vi "pass new incidents onto the network stream.vi"(7 "RT Queues":T1, 8 "Comms data":T2={"Parameters"={"error writer name"="error writer", "command reader name"="command reader", "error buffer size"=16, "command buffer size"=16, "scanivalveIP"="", "scanivalvePeriod"=16}, "Variables"={"listen schedule"=0, "incident buffer"=[], "command stream"="", "error stream"="", "waiting for command stream connect"=FALSE, "waiting for error stream connect"=FALSE, "scanivalve connection"=refnum, "scanivalveScheduleID"=16}}, 10 "incident":variant) -> (0 "Comms data out":T2={"Parameters"={"error writer name"="error writer", "command reader name"="command reader", "error buffer size"=16, "command buffer size"=16, "scanivalveIP"="", "scanivalvePeriod"=16}, "Variables"={"listen schedule"=0, "incident buffer"=[], "command stream"="", "error stream"="", "waiting for command stream connect"=FALSE, "waiting for error stream connect"=FALSE, "scanivalve connection"=refnum, "scanivalveScheduleID"=16}}, 2 "buffered messages":i32)   [LabVIEW 2018]
uses:
  comms data.ctl
  Type Defs/generic incident.ctl
  Type Defs/Queues cluster.ctl
  Chris VIs/Message Scheduler/message scheduler.lvclass
  Queue VIs/En-queue RT comms element.vi
  <resource>/objmgr/ni.dex.rc
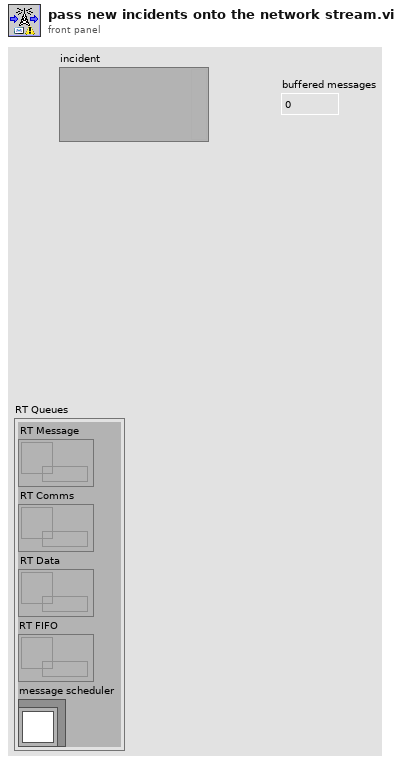
[diagram p1: front panel]
types:
  T1 = typedef "Queues cluster.ctl" = cluster{"RT Message":refnum<queue>, "RT Comms":refnum<queue>, "RT Data":refnum<queue>, "RT FIFO":refnum<queue>, "message scheduler":refnum<class "message scheduler.lvclass">}
  T2 = typedef "comms data.ctl" = cluster{"Parameters":cluster{"error writer name":string, "command reader name":string, "error buffer size":i32, "command buffer size":i32, "scanivalveIP":string, "scanivalvePeriod":u16}, "Variables":cluster{"listen schedule":u32, "incident buffer":T3[], "command stream":refnum<k21>, "error stream":refnum<k21>, "waiting for command stream connect":bool, "waiting for error stream connect":bool, "scanivalve connection":refnum<k5>, "scanivalveScheduleID":u32}}
  T3 = typedef "generic incident.ctl" = cluster{"timestamp":timestamp, "type":string, "Variant":variant}
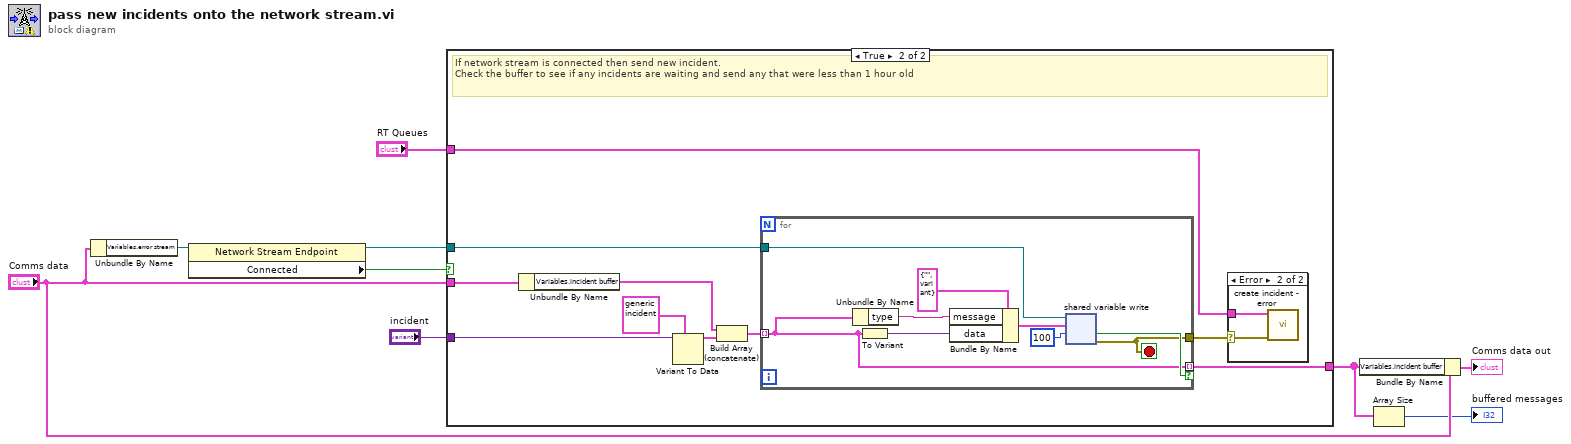
[diagram p0: block diagram]
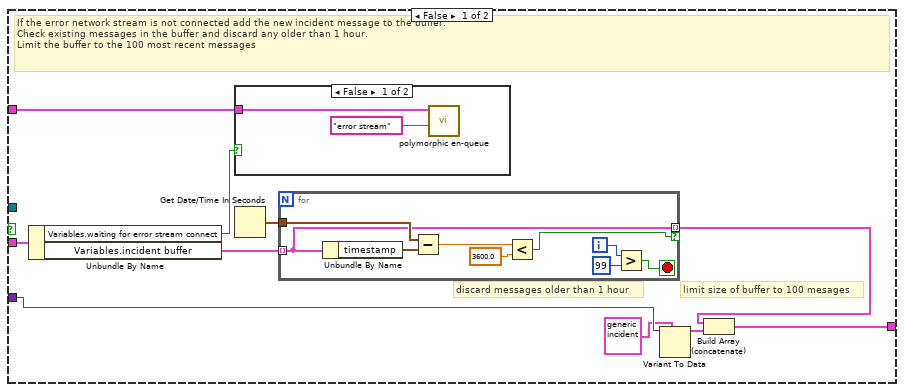
[diagram p2: hidden frame]
diagram:
  n1 = Unbundle By Name("Comms data") -> ("Variables.error stream"=w9:refnum<k21>)
  n2 = property class="Network Stream Endpoint"(reference=w9) -> (reference out=w8:refnum<k21>, "Connected"=w7:bool)  [unwired: 1 in, 1 out]
  n3 = case shown="True" w7 {
    tunnel: w8 -> [_ w34]
    tunnel: "incident" -> [w16 w39]
    tunnel: "Comms data" -> [w18 w40]
    tunnel: [w12 w33] -> w2
    tunnel: "RT Queues" -> [w11 w31]
    frame False {
      # "discard messages older than 1 hour"
      # "limit size of buffer to 100 mesages"
      # "If the error network stream is not connected add the new incident message to the buffer.\nCheck existing messages in the buffer and discard any older than 1 hour.\nLimit the buffer to the 100 most recent messages"
      n4 = Unbundle By Name(w18) -> ("Variables.waiting for error stream connect"=w10:bool, "Variables.incident buffer"=w17:T3[])
      n5 = case shown="False" w10 {
        tunnel: w11 -> [w21 _]
        frame False {
          n6 = call-poly "polymorphic en-queue.vi"("Message"="error stream", "RT Queues"=w21) -> ()  [unwired: 9 in, 1 out]
        }
        frame True {
        }
      }
      n7 = Get Date/Time In Seconds() -> (seconds since 1Jan1904=w19:timestamp)
      n8 = for {
        tunnel: w19 -> [w28]
        tunnel: w17 -> [w23] mode=indexing
        tunnel: [w23] -> w13 mode=indexing if=w22
        i -> [w27]
        stop <- w25 stop-if-true
        n9 = Unbundle By Name(w23) -> ("timestamp"=w24:timestamp)
        n10 = Subtract(x=w28, y=w24) -> (x-y=w30:dbl)
        n11 = Less?(x=w30, y=3600.0) -> (x < y?=w22:bool)
        n12 = Greater?(x=w27, y=99) -> (0:w25:bool)
      }
      n13 = Variant To Data(type=T3 {"timestamp"=timestamp(0 s since 1904-01-01), "type"="", "Variant"=variant} ("incident cluster"), Variant=w16) -> (data=w14:T3)  [unwired: 1 in, 1 out]
      n14 = Build Array (concatenate)(w13, w14) -> (w12:T3[])
    }
    frame True {
      # "If network stream is connected then send new incident.\nCheck the buffer to see if any incidents are waiting and send any that were less than 1 hour old"
      n15 = Unbundle By Name(w40) -> ("Variables.incident buffer"=w37:T3[])
      n16 = Variant To Data(type=T3 {"timestamp"=timestamp(0 s since 1904-01-01), "type"="", "Variant"=variant} ("incident cluster"), Variant=w39) -> (data=w36:T3)  [unwired: 1 in, 1 out]
      n17 = Build Array (concatenate)(w37, w36) -> (w35:T3[])
      n18 = for {
        tunnel: w35 -> [w44] mode=indexing
        tunnel: w34 -> [w50]
        tunnel: [w44] -> w33 mode=indexing if=w46
        tunnel: [w45] -> w32
        stop <- w45 stop-if-true
        n19 = Unbundle By Name(w44) -> ("type"=w43:string)
        n20 = To Variant(anything=w44) -> (Variant=w51:variant)
        n21 = Bundle By Name(cluster=cluster{"message":string, "data":variant} {"message"="", "data"=variant} ("data in"), "message"=w43, "data"=w51) -> (w48:cluster{"message":string, "data":variant})
        n22 = shared-variable-write(w50, w48, 100 ("timeout ms (-1)")) -> (w45:errorcluster, w46:bool)  [unwired: 1 in, 1 out]
      }
      n23 = case shown="Error" w32 {
        selector: w32 -> [_ w42]
        tunnel: w31 -> [_ w41]
        frame No Error {
        }
        frame Error {
          n24 = call "create incident - error.vi"("error"=w42, "RT Queues"=w41) -> ()  [unwired: 9 in, 1 out]
        }
      }
    }
  }
  n25 = Bundle By Name(cluster="Comms data", "Variables.incident buffer"=w2) -> (→"Comms data out":T2)
  n26 = Array Size(array=w2) -> (size(s)=→"buffered messages":i32)
